vi "Test path.vi"() -> ()   [LabVIEW 2015]
uses:
  <vilib>/Utility/sysdir.llb/System Directory Type.ctl
  Mag Lab Root/Mag Lab Root.lvclass/Mag Lab Root.ctl
  Hardware/Mag Lab Hardware.lvclass
  Mag Lab Root/Mag Lab Root.lvclass
panel:
  out "Array":string[](array[string])
  out "appended path":path
  out "error out":errorcluster
  out "VI Path":path
  out "Application Directory":path
  in  "system directory type":T1 items=["User Home"=0, "User Desktop"=1, "User Documents"=2, "User Application Data"=3, "User Preferences"=4, "User Temporary"=5, "Public Documents"=6, "Public Application Data"=7, "Public Preferences"=8, "Public Cache"=13, "System Core Libraries"=9, "System Installed Libraries"=10, "Application Files"=11, "Boot Volume Root"=12]
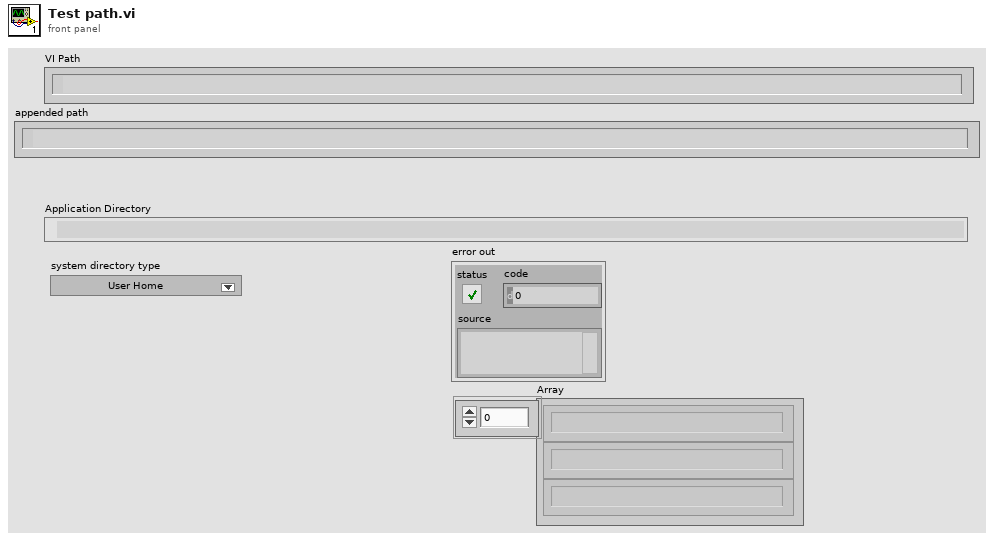
[diagram p1: front panel]
types:
  T1 = typedef "System Directory Type.ctl" = i32
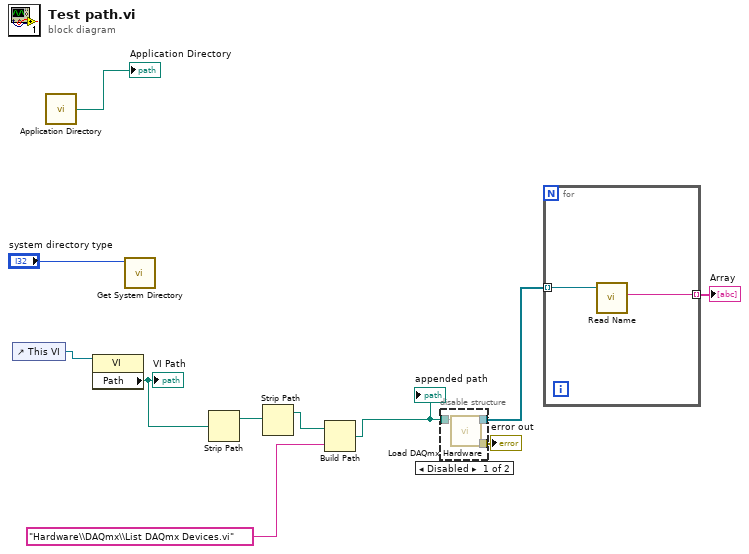
[diagram p0: block diagram]
diagram:
  n1 = control-ref of="This VI"() -> (w9:refnum<vi>)
  n2 = call <vilib>:"Application Directory.vi"() -> ("Application Directory"=→"Application Directory":path)
  n3 = property class="VI"(reference=w9) -> ("Path"=w8:path)  [unwired: 1 in, 2 out]
  "VI Path" <- w8
  n4 = call <vilib>:"Get System Directory.vi"("system directory type"="system directory type") -> ()  [unwired: 10 in, 1 out]
  n5 = Strip Path(path=w8) -> (stripped path=w7:path)  [unwired: 1 out]
  n6 = Strip Path(path=w7) -> (stripped path=w6:path)  [unwired: 1 out]
  n7 = Build Path(base path=w6, name or relative path="Hardware\\DAQmx\\List DAQmx Devices.vi") -> (appended path=w4:path)
  "appended path" <- w4
  n8 = disable-structure shown="Disabled" {
    disable-tunnel: w4 -> [w14 _]
    disable-tunnel: [w13 _] -> w3
    disable-tunnel: [w12 _] -> w2
    frame Disabled {
      n9 = call "Load DAQmx Hardware.vi"("vi path"=w14) -> ("error out"=w13:errorcluster, "DAQmx Devices"=w12:refnum<class "Mag Lab Hardware.lvclass">[])  [unwired: 9 in]
    }
    frame Enabled {
    }
  }
  "error out" <- w3
  n10 = for {
    tunnel: w2 -> [w16] mode=indexing
    tunnel: [w15] -> w1 mode=indexing
    n11 = call "Read Name.vi"("Mag Lab Root in"=w16) -> ("Name"=w15:string)  [unwired: 8 in, 2 out]
  }
  "Array" <- w1
